vi "DLPVA_4_WriteAll.vi"(0 "Gain (dB)":dbl, 5 "Gain_1o":bool, 7 "Gain_2 o":bool, 9 "AC/DC o":bool, 11 "Filter o":bool) -> ()   [LabVIEW 2013]
panel:
  # "4"
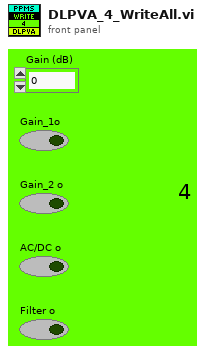
[diagram p1: front panel]
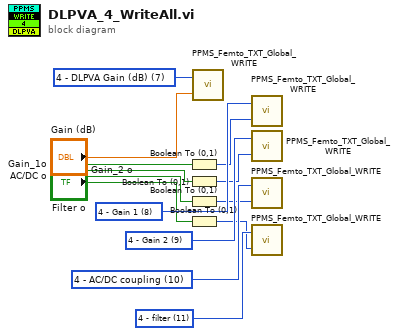
[diagram p0: block diagram]
diagram:
  w11 = u16 11 items=["1 - DDPCA Gain (V/A)", "2 - DDPCA Gain (V/A)", "3 - DLPVA Gain (dB)", "3 - Gain 1", "3 - Gain 2", "3 - AC/DC coupling", "3 - filter", "4 - DLPVA Gain (dB)", "4 - Gain 1", "4 - Gain 2", "4 - AC/DC coupling", "4 - filter"] ("Property")
  w12 = u16 10 items=["1 - DDPCA Gain (V/A)", "2 - DDPCA Gain (V/A)", "3 - DLPVA Gain (dB)", "3 - Gain 1", "3 - Gain 2", "3 - AC/DC coupling", "3 - filter", "4 - DLPVA Gain (dB)", "4 - Gain 1", "4 - Gain 2", "4 - AC/DC coupling", "4 - filter"] ("Property")
  w13 = u16 9 items=["1 - DDPCA Gain (V/A)", "2 - DDPCA Gain (V/A)", "3 - DLPVA Gain (dB)", "3 - Gain 1", "3 - Gain 2", "3 - AC/DC coupling", "3 - filter", "4 - DLPVA Gain (dB)", "4 - Gain 1", "4 - Gain 2", "4 - AC/DC coupling", "4 - filter"] ("Property")
  w14 = u16 8 items=["1 - DDPCA Gain (V/A)", "2 - DDPCA Gain (V/A)", "3 - DLPVA Gain (dB)", "3 - Gain 1", "3 - Gain 2", "3 - AC/DC coupling", "3 - filter", "4 - DLPVA Gain (dB)", "4 - Gain 1", "4 - Gain 2", "4 - AC/DC coupling", "4 - filter"] ("Property")
  w10 = u16 7 items=["1 - DDPCA Gain (V/A)", "2 - DDPCA Gain (V/A)", "3 - DLPVA Gain (dB)", "3 - Gain 1", "3 - Gain 2", "3 - AC/DC coupling", "3 - filter", "4 - DLPVA Gain (dB)", "4 - Gain 1", "4 - Gain 2", "4 - AC/DC coupling", "4 - filter"] ("Property")
  n1 = Boolean To (0,1)(Boolean="Gain_1o") -> (0, 1=w1:i16)
  n2 = Boolean To (0,1)(Boolean="Gain_2 o") -> (0, 1=w4:i16)
  n3 = Boolean To (0,1)(Boolean="AC/DC o") -> (0, 1=w3:i16)
  n4 = Boolean To (0,1)(Boolean="Filter o") -> (0, 1=w2:i16)
  n5 = call "PPMS_Femto_TXT_Global_WRITE.vi"("Value"="Gain (dB)", "Property"=w10) -> ()  [unwired: 2 in]
  n6 = call "PPMS_Femto_TXT_Global_WRITE.vi"("Value"=w1, "Property"=w14) -> ()  [unwired: 2 in]
  n7 = call "PPMS_Femto_TXT_Global_WRITE.vi"("Value"=w4, "Property"=w13) -> ()  [unwired: 2 in]
  n8 = call "PPMS_Femto_TXT_Global_WRITE.vi"("Value"=w3, "Property"=w12) -> ()  [unwired: 2 in]
  n9 = call "PPMS_Femto_TXT_Global_WRITE.vi"("Value"=w2, "Property"=w11) -> ()  [unwired: 2 in]
